vi "Perform Current Gain.vi"(6 "error in":errorcluster, 8 "MaxRead":i32, 9 "Channel in":u16) -> (0 "error out":errorcluster, 1 "Messages":T1(array[cluster]), 2 "Pass":bool, 3 "Channel out":u16)   [LabVIEW 2023]
uses:
  7e6a34f5-6666-41a7-b638-f367e94293a1.vi
  Communication/PCAN2023/PCAN API.lvlib
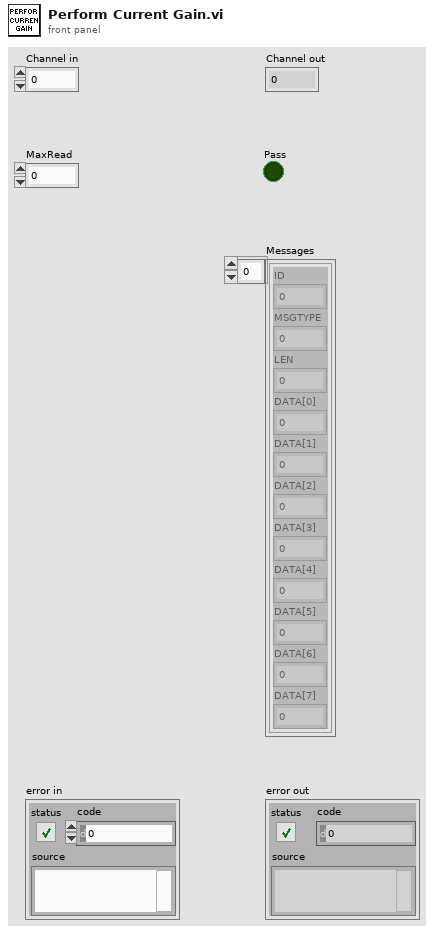
[diagram p1: front panel]
types:
  T1 = cluster{"ID":u32, "MSGTYPE":u8, "LEN":u8, "DATA[0]":u8, "DATA[1]":u8, "DATA[2]":u8, "DATA[3]":u8, "DATA[4]":u8, "DATA[5]":u8, "DATA[6]":u8, "DATA[7]":u8}[]
  T2 = cluster{"ID":u32, "MSGTYPE":u8, "LEN":u8, "DATA[0]":u8, "DATA[1]":u8, "DATA[2]":u8, "DATA[3]":u8, "DATA[4]":u8, "DATA[5]":u8, "DATA[6]":u8, "DATA[7]":u8}
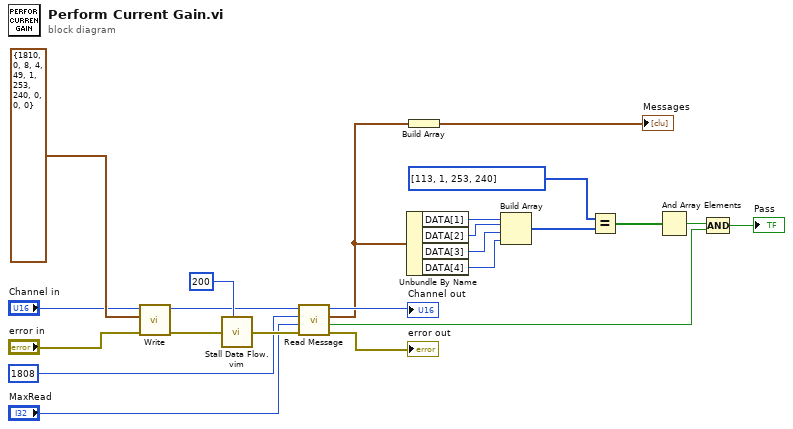
[diagram p0: block diagram]
diagram:
  n1 = call "Write.vi"("error in"="error in", "MessageBuffer"=T2 {"ID"=1810, "MSGTYPE"=0, "LEN"=8, "DATA[0]"=4, "DATA[1]"=49, "DATA[2]"=1, "DATA[3]"=253, "DATA[4]"=240, "DATA[5]"=0, "DATA[6]"=0, "DATA[7]"=0}, "Channel"="Channel in") -> ("error out"=w22:errorcluster, "Channel out"=w8:u16)  [unwired: 5 in, 2 out]
  n2 = call "Stall Data Flow.vim"("value in"=w22, "milliseconds to wait"=u32 200) -> ("value out"=w6:errorcluster)  [unwired: 1 out]
  n3 = call "Read Message.vi"("error in"=w6, "MaxRead"="MaxRead", "ID"=u32 1808, "Channel in"=w8) -> ("error out"=→"error out":errorcluster, "Passed"=w2:bool, "Last Message"=w1:T2, "Channel out"=→"Channel out":u16)  [unwired: 3 in, 1 out]
  n4 = Unbundle By Name(w1) -> ("DATA[1]"=w15:u8, "DATA[2]"=w14:u8, "DATA[3]"=w13:u8, "DATA[4]"=w12:u8)
  n5 = Build Array(w1) -> (→"Messages":T1)
  n6 = Build Array(w15, w14, w13, w12) -> (w11:u8[])
  n7 = Equal?(x=u8[] [113, 1, 253, 240], y=w11) -> (x = y?=w10:bool[])
  n8 = And Array Elements(Boolean array=w10) -> (logical AND=w9:bool)
  n9 = Compound Arithmetic op=AND(w9, w2) -> (→"Pass":bool)
